vi "Get Cal Func List.vi"(6 "참조":refnum<vi>, 8 "error in (no error)":errorcluster caption="에러 입력(에러 없음)") -> (0 "error out":errorcluster caption="에러 출력", 1 "Func List":string[][](array[string]))   [LabVIEW 2020]
uses:
  Controls/Clst_Query Info.ctl
  Controls/Cmd_Read Query.ctl
  Variables/Global_Cal Info.vi
  Public/Polymorph/Array Dedup_2D Str.vi
  <vilib>/Utility/error.llb/Error Cluster From Error Code.vi
  <vilib>/ErrorRing/Error Ring.xnode
  <vilib>/addons/database/NI_Database_API.lvlib
panel:
  out "옵션":string
  out "형식":string
  out "세부분류코드":string
  out "Cal Func List":string[][](array[string])
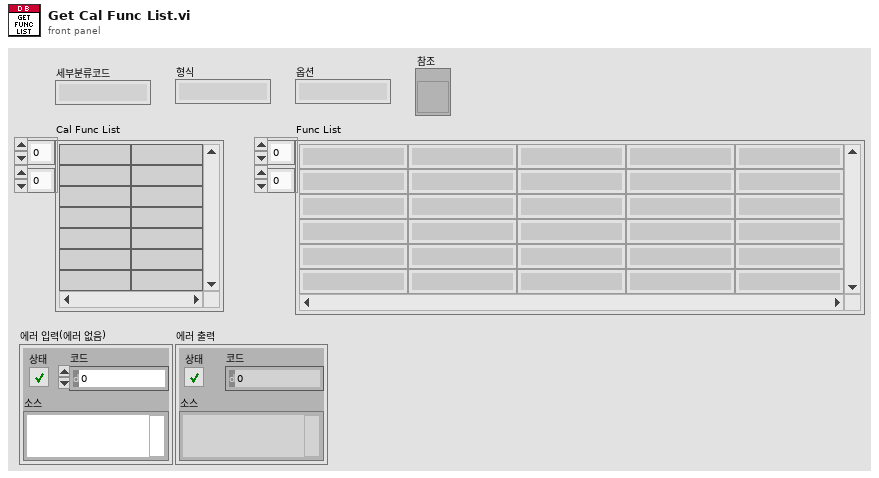
[diagram p1: front panel]
types:
  T1 = typedef "Cmd_Read Query.ctl" = enum16{"교정자 이름 얻기", "인증교정자 얻기", "기술책임자 얻기", "기책부책 얻기", "등록번호 얻기", "등록정보 얻기", "업체정보 얻기", "교정일자(CAMAS) 얻기", "교정일자(CALSTD) 얻기", "교정환경 얻기", "교정절차서 목록 얻기", "교정절차서명 얻기", "교정절차 목록얻기", "교정절차 얻기", "PROC 교정절차 얻기", "PROC SPEC 얻기", "교정절차(Func별) 얻기", "교정절차(Func_ext별) 얻기", "기관코드 얻기", "교정기능(세부분류) 얻기", "교정기능(모델) 얻기", "교정기능 목록 얻기", "교정기능 명칭 얻기", "교정기능 항목명칭 얻기", "DB (사용기준기) 얻기", "DB (기준기이름) 얻기", "DB (기준기이름목록) 얻기", "DB (기준기목록) 얻기", "DB (기준기값) 얻기", "DB (CMC) 얻기", "DB (FUNC) 얻기", "DB (CALNAME) 얻기", "DB (STDNAME) 얻기", "DB (SPEC) 얻기", "모델(항목전체) 얻기", "모델(최대범위) 얻기", "모델(최소범위) 얻기", "모델(최대최소) 얻기", "모델(범위조건) 얻기", "모델(등록요청) 얻기", "모델(형식별) 얻기", "모델(조건별) 얻기", "모델(모델검색) 얻기", "세부분류 목록 얻기", "기준기등록리스트 얻기", "STD Cal Date Check", "DB등록일자 얻기", "적용항목 얻기", "기타정보 얻기", "기준기요청 얻기", "서버버전 얻기"}
  T2 = typedef "Clst_Query Info.ctl" = cluster{"사번":string, "등록번호":string, "업체명":string, "세부분류코드":string, "형식":string, "기기번호":string, "FUNC":string, "FUNC_EXT":string, "옵션":string, "추가문자열":string, "일자":string, "배열 1":string[], "배열 2":string[], "항목명":string, "문자열":string, "이름":string}
  T3 = cluster{"세부분류코드":string, "형식":string, "옵션":string, "측정기명":string, "EXCEL파일명":string, "TEMP":string}
  T4 = typedef "NI_Database_API.lvlib/Conn ObjectReference.ctl" = refnum<k1>
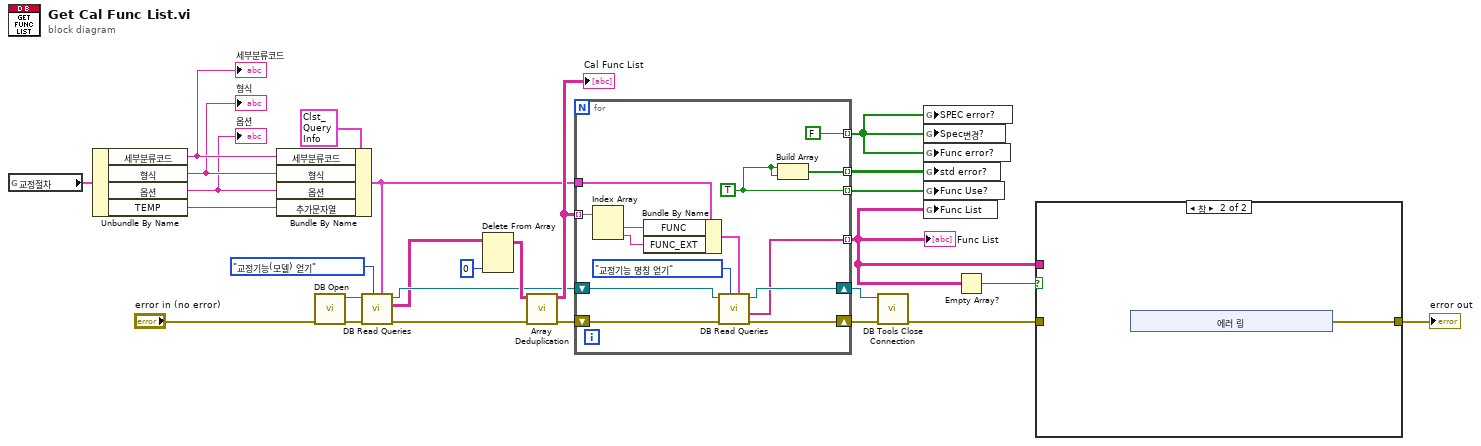
[diagram p0: block diagram]
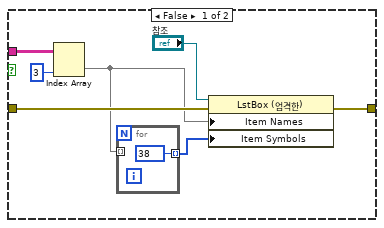
[diagram p2: hidden frame]
diagram:
  n1 = global read "Global_Cal Info.vi" "교정절차"() -> (w23:T3)
  n2 = Unbundle By Name(w23) -> ("세부분류코드"=w22:string, "형식"=w18:string, "옵션"=w17:string, "TEMP"=w5:string)
  "세부분류코드" <- w22
  "형식" <- w18
  "옵션" <- w17
  n3 = Bundle By Name(cluster=T2 {"사번"="", "등록번호"="", "업체명"="", "세부분류코드"="", "형식"="", "기기번호"="", "FUNC"="", "FUNC_EXT"="", "옵션"="", "추가문자열"="", "일자"="", "배열 1"=[], "배열 2"=[], "항목명"="", "문자열"="", "이름"=""} ("Query info"), "세부분류코드"=w22, "형식"=w18, "옵션"=w17, "추가문자열"=w5) -> (w2:T2)
  n4 = call "DB Open.vi"("에러 입력"="error in (no error)") -> ("에러 출력"=w26:errorcluster, "참조 번호 출력"=w25:T4)  [unwired: 9 in]
  n5 = call "DB Read Queries.vi"("Query info"=w2, "Query Command"=Cmd_Read_Query."교정기능(모델) 얻기", "에러 입력(에러 없음)"=w26, "참조 번호 입력"=w25) -> ("에러 출력"=w9:errorcluster, "Data"=w6:string[][], "참조 번호 출력"=w8:T4)  [unwired: 3 in, 2 out]
  n6 = Delete From Array(array=w6, index (col)=0 ("비활성화된 인덱스 (열)")) -> (array with subset deleted=w13:string[][])  [unwired: 2 in, 1 out]
  n7 = call-poly "Array Deduplication.vi"("error in (no error)"=w9, "배열 in"=w13) -> ("error out"=w21:errorcluster, "배열 out"=w12:string[][])  [unwired: 8 in]
  "Cal Func List" <- w12
  n8 = for {
    tunnel: w12 -> [w35] mode=indexing
    shift-right: [w40] -> w20
    shift-left: w21 -> [w41]
    shift-right: [w36] -> w19
    shift-left: w8 -> [w38]
    tunnel: [w32] -> w4 mode=indexing
    tunnel: [w31] -> w11 mode=indexing
    tunnel: [w30] -> w10 mode=indexing
    tunnel: [FALSE] -> w1 mode=indexing
    tunnel: w2 -> [w29]
    w31 = TRUE
    n9 = Index Array(array=w35) -> (element #1=w34:string, element #2=w33:string)  [unwired: 2 in]
    n10 = Bundle By Name(cluster=w29, "FUNC"=w34, "FUNC_EXT"=w33) -> (w37:T2)
    n11 = call "DB Read Queries.vi"("Query info"=w37, "Query Command"=Cmd_Read_Query."교정기능 명칭 얻기", "에러 입력(에러 없음)"=w41, "참조 번호 입력"=w38) -> ("에러 출력"=w40:errorcluster, "Data (0번행)"=w32:string[], "참조 번호 출력"=w36:T4)  [unwired: 3 in, 2 out]
    n12 = Build Array(w31, w31) -> (w30:bool[])
  }
  "Func List" <- w4
  n13 = call <vilib>:"DB Tools Close Connection.vi"("error in (no error)"=w20, "connection reference"=w19) -> ("error out"=w16:errorcluster)  [unwired: 5 in]
  n14 = global write "Global_Cal Info.vi" "SPEC error?"(w1) -> ()
  n15 = global write "Global_Cal Info.vi" "Spec변경?"(w1) -> ()
  n16 = global write "Global_Cal Info.vi" "Func error?"(w1) -> ()
  n17 = global write "Global_Cal Info.vi" "std error?"(w10) -> ()
  n18 = global write "Global_Cal Info.vi" "Func Use?"(w11) -> ()
  n19 = global write "Global_Cal Info.vi" "Func List"(w4) -> ()
  n20 = Empty Array?(array=w4) -> (empty?=w3:bool)
  n21 = case shown="참" w3 {
    tunnel: w4 -> [w47 _]
    tunnel: w16 -> [w46 _]
    tunnel: [w45 w50] -> w15
    frame False {
      n22 = Index Array(array=w47, index (col)=3 ("비활성화된 인덱스 (열)")) -> (element=w43:string[])  [unwired: 1 in]
      n23 = for {
        tunnel: w43 -> [_] mode=indexing
        tunnel: [38] -> w42 mode=indexing
      }
      n24 = property on="프로퍼티 노드" class="LstBox (엄격한)"(reference="참조", error in=w46, "Item Names"=w43, "Item Symbols"=w42) -> (error out=w45:errorcluster)  [unwired: 1 out]
    }
    frame True {
      n25 = xnode "에러 링"() -> ("에러 출력"=w50:errorcluster)
    }
  }
  "error out" <- w15
